vi "ascii_textfilter.vi"(11 "Inputstring":string) -> (3 "Outputstring":string)   [LabVIEW 2013]
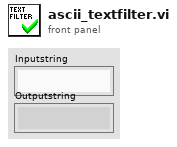
[diagram p1: front panel]
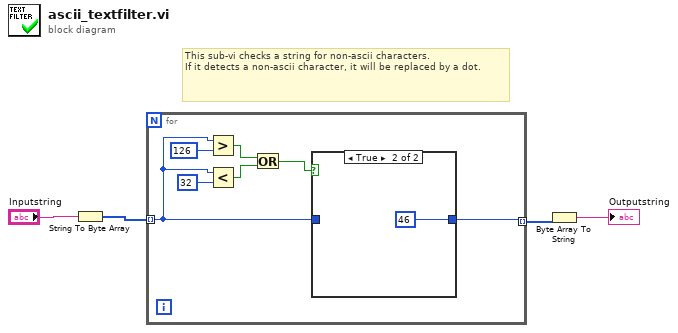
[diagram p0: block diagram]
diagram:
  # "This sub-vi checks a string for non-ascii characters.\nIf it detects a non-ascii character, it will be replaced by a dot."
  n1 = String To Byte Array(string="Inputstring") -> (unsigned byte array=w2:u8[])
  n2 = for {
    tunnel: w2 -> [w5] mode=indexing
    tunnel: [w7] -> w1 mode=indexing
    n3 = Greater?(x=w5, y=u8 126 ("x")) -> (0:w9:bool)
    n4 = Less?(x=w5, y=u8 32) -> (x < y?=w10:bool)
    n5 = Or(x=w9, y=w10) -> (x .or. y?=w8:bool)
    n6 = case shown="True" w8 {
      tunnel: w5 -> [w12 _]
      tunnel: [w12 46] -> w7
      frame False {
      }
      frame True {
      }
    }
  }
  n7 = Byte Array To String(unsigned byte array=w1) -> (string=→"Outputstring":string)
